vi "App - analyze RUS V6.vi"() -> ()   [LabVIEW 2018] (continued)
"radius"=0.4754648959407264}}, "timestamp(min)"=862.4166666641831, "timestamp"=timestamp(3493779566 s since 1904-01-01), "Magn Field(T)"=0.0}, {"temperature"=77.512, "lorentzian"={"A (VHz)"=0.00029695540647974435, "f (Hz)"=665.0338682665438, "G (Hz)"=0.032873121586090105, "phi(rad)"=3.411171742356422, "Q"=20230.323017085953, "Norm  Ampl"=0.015527303955909932, "bg (V)"=0.1217964163037196-0.45928093647211954i, "4corners"={"z (-pi/2)"=-0.45928093647211954-0.1297964163037196i, "z(inf)"=0.1217964163037196-0.45928093647211954i, "z (pi/2)"=0.45128093647211953+0.1217964163037196i, "z center"=-0.0040000000000000036-0.0040000000000000036i, "z(0)"=-0.1297964163037196+0.45128093647211953i, "radius"=0.4723404169344276}}, "timestamp(min)"=863.75, "timestamp"=timestamp(3493779646 s since 1904-01-01), "Magn Field(T)"=0.0}, {"temperature"=77.434, "lorentzian"={"A (VHz)"=0.0002808833623249405, "f (Hz)"=665.0132269511125, "G (Hz)"=0.030053559356176034, "phi(rad)"=3.2164772260932604, "Q"=22127.602892881696, "Norm  Ampl"=0.014704545280424244, "bg (V)"=0.05660513936673565-0.4919067745838443i, "4corners"={"z (-pi/2)"=-0.4679067745838443-0.04060513936673563i, "z(inf)"=0.05660513936673565-0.4919067745838443i, "z (pi/2)"=0.5079067745838444+0.032605139366735626i, "z center"=0.020000000000000018-0.0040000000000000036i, "z(0)"=-0.016605139366735612+0.4839067745838443i, "radius"=0.4892779955330797}}, "timestamp(min)"=865.0666666701436, "timestamp"=timestamp(3493779725 s since 1904-01-01), "Magn Field(T)"=0.0}, {"temperature"=77.354, "lorentzian"={"A (VHz)"=0.00024324022719169407, "f (Hz)"=664.9933134080237, "G (Hz)"=0.02605319858686614, "phi(rad)"=3.1017031738643666, "Q"=25524.440355790255, "Norm  Ampl"=0.01188779498495909, "bg (V)"=0.04180368485342219-0.49192630188829584i, "4corners"={"z (-pi/2)"=-0.3959263018882958-0.01780368485342211i, "z(inf)"=0.04180368485342219-0.49192630188829584i, "z (pi/2)"=0.5159263018882959-0.05419631514657784i, "z center"=0.06000000000000005-0.035999999999999976i, "z(0)"=0.07819631514657792+0.4199263018882959i, "radius"=0.4562892707904176}}, "timestamp(min)"=866.3833333328366, "timestamp"=timestamp(3493779804 s since 1904-01-01), "Magn Field(T)"=0.0}, {"temperature"=77.279, "lorentzian"={"A (VHz)"=0.0002767684428284637, "f (Hz)"=664.9763291448037, "G (Hz)"=0.03131222664140858, "phi(rad)"=3.3392624127704833, "Q"=21236.954393572625, "Norm  Ampl"=0.014856092973334787, "bg (V)"=0.09717490852872655-0.47721119114295873i, "4corners"={"z (-pi/2)"=-0.4612111911429587-0.10517490852872656i, "z(inf)"=0.09717490852872655-0.47721119114295873i, "z (pi/2)"=0.46921119114295873+0.08117490852872654i, "z center"=0.0040000000000000036-0.01200000000000001i, "z(0)"=-0.08917490852872655+0.4532111911429587i, "radius"=0.4744502249382827}}, "timestamp(min)"=867.7166666686535, "timestamp"=timestamp(3493779884 s since 1904-01-01), "Magn Field(T)"=0.0}, {"temperature"=77.2, "lorentzian"={"A (VHz)"=0.00025465138660872073, "f (Hz)"=664.9564180576857, "G (Hz)"=0.02920076503699602, "phi(rad)"=3.2865495056553193, "Q"=22771.883449464993, "Norm  Ampl"=0.013732392409333284, "bg (V)"=0.07193111188153918-0.4693429105783114i, "4corners"={"z (-pi/2)"=-0.4613429105783114-0.07193111188153918i, "z(inf)"=0.07193111188153918-0.4693429105783114i, "z (pi/2)"=0.4693429105783114+0.06393111188153917i, "z center"=0.0040000000000000036-0.0040000000000000036i, "z(0)"=-0.06393111188153917+0.4613429105783114i, "radius"=0.470275090119556}}, "timestamp(min)"=869.0333333313465, "timestamp"=timestamp(3493779963 s since 1904-01-01), "Magn Field(T)"=0.0}, {"temperature"=77.118, "lorentzian"={"A (VHz)"=0.00027838491301398664, "f (Hz)"=664.9357800881095, "G (Hz)"=0.03181971997495915, "phi(rad)"=3.269604239812998, "Q"=20896.971457052023, "Norm  Ampl"=0.015065275703701596, "bg (V)"=0.06444261324766684-0.48158323658272556i, "4corners"={"z (-pi/2)"=-0.46558323658272555-0.07244261324766685i, "z(inf)"=0.06444261324766684-0.48158323658272556i, "z (pi/2)"=0.47358323658272555+0.048442613247666834i, "z center"=0.0040000000000000036-0.01200000000000001i, "z(0)"=-0.05644261324766684+0.45758323658272554i, "radius"=0.4734572056434615}}, "timestamp(min)"=870.3500000014901, "timestamp"=timestamp(3493780042 s since 1904-01-01), "Magn Field(T)"=0.0}, {"temperature"=77.043, "lorentzian"={"A (VHz)"=0.00025512847575077615, "f (Hz)"=664.9153463888829, "G (Hz)"=0.028245509163786278, "phi(rad)"=3.1126571502773475, "Q"=23540.568609801325, "Norm  Ampl"=0.013385825226800704, "bg (V)"=0.022289093204638705-0.5017114778047216i, "4corners"={"z (-pi/2)"=-0.43771147780472147-0.0142890932046387i, "z(inf)"=0.022289093204638705-0.5017114778047216i, "z (pi/2)"=0.5097114778047216-0.04171090679536135i, "z center"=0.03600000000000003-0.028000000000000025i, "z(0)"=0.04971090679536136+0.4457114778047215i, "radius"=0.4739098576407587}}, "timestamp(min)"=871.683333337307, "timestamp"=timestamp(3493780122 s since 1904-01-01), "Magn Field(T)"=0.0}, {"temperature"=76.965, "lorentzian"={"A (VHz)"=0.000290950002143314, "f (Hz)"=664.8962985459169, "G (Hz)"=0.033622915172790445, "phi(rad)"=3.3360289701037327, "Q"=19775.09371596632, "Norm  Ampl"=0.015800250307514467, "bg (V)"=0.08679586668019772-0.47307013478150894i, "4corners"={"z (-pi/2)"=-0.46507013478150894-0.10279586668019773i, "z(inf)"=0.08679586668019772-0.47307013478150894i, "z (pi/2)"=0.45707013478150893+0.07879586668019771i, "z center"=-0.0040000000000000036-0.01200000000000001i, "z(0)"=-0.09479586668019772+0.4490701347815089i, "radius"=0.4699250563586146}}, "timestamp(min)"=873.0, "timestamp"=timestamp(3493780201 s since 1904-01-01), "Magn Field(T)"=0.0}, {"temperature"=76.89, "lorentzian"={"A (VHz)"=0.00027920835625752665, "f (Hz)"=664.877249248592, "G (Hz)"=0.03212210537837073, "phi(rad)"=3.306412896473442, "Q"=20698.433101345967, "Norm  Ampl"=0.015111162714631697, "bg (V)"=0.06518560735297112-0.4760534616565365i, "4corners"={"z (-pi/2)"=-0.4760534616565365-0.08918560735297114i, "z(inf)"=0.06518560735297112-0.4760534616565365i, "z (pi/2)"=0.4520534616565365+0.06518560735297112i, "z center"=-0.01200000000000001-0.01200000000000001i, "z(0)"=-0.08918560735297114+0.4520534616565365i, "radius"=0.470428775967055}}, "timestamp(min)"=874.3333333358169, "timestamp"=timestamp(3493780281 s since 1904-01-01), "Magn Field(T)"=0.0}, {"temperature"=76.811, "lorentzian"={"A (VHz)"=0.0002809182349613738, "f (Hz)"=664.8577998829521, "G (Hz)"=0.03227972899383772, "phi(rad)"=3.326321935294232, "Q"=20596.75903753328, "Norm  Ampl"=0.01526280982428019, "bg (V)"=0.09084953461030412-0.4767848365941506i, "4corners"={"z (-pi/2)"=-0.4607848365941506-0.09884953461030413i, "z(inf)"=0.09084953461030412-0.4767848365941506i, "z (pi/2)"=0.4687848365941506+0.07484953461030411i, "z center"=0.0040000000000000036-0.01200000000000001i, "z(0)"=-0.08284953461030412+0.4527848365941506i, "radius"=0.47282955278818783}}, "timestamp(min)"=875.6499999985099, "timestamp"=timestamp(3493780360 s since 1904-01-01), "Magn Field(T)"=0.0}, {"temperature"=76.733, "lorentzian"={"A (VHz)"=0.0002685357531772652, "f (Hz)"=664.8386786299899, "G (Hz)"=0.031013359018924134, "phi(rad)"=3.3158635131911067, "Q"=21437.170937347033, "Norm  Ampl"=0.014446963332719644, "bg (V)"=0.07677036203873196-0.4707745055716542i, "4corners"={"z (-pi/2)"=-0.46277450557165417-0.09277036203873197i, "z(inf)"=0.07677036203873196-0.4707745055716542i, "z (pi/2)"=0.45477450557165416+0.06877036203873195i, "z center"=-0.0040000000000000036-0.01200000000000001i, "z(0)"=-0.08477036203873196+0.44677450557165416i, "radius"=0.46583033214506714}}, "timestamp(min)"=876.9666666686535, "timestamp"=timestamp(3493780439 s since 1904-01-01), "Magn Field(T)"=0.0}, {"temperature"=76.659, "lorentzian"={"A (VHz)"=0.00027897248558761146, "f (Hz)"=664.8188133493377, "G (Hz)"=0.03153421429238599, "phi(rad)"=3.3051331613850907, "Q"=21082.460060210215, "Norm  Ampl"=0.014924965616204034, "bg (V)"=0.08105823087278374-0.4789792025319606i, "4corners"={"z (-pi/2)"=-0.46297920253196057-0.08905823087278375i, "z(inf)"=0.08105823087278374-0.4789792025319606i, "z (pi/2)"=0.4709792025319606+0.06505823087278373i, "z center"=0.0040000000000000036-0.01200000000000001i, "z(0)"=-0.07305823087278374+0.45497920253196056i, "radius"=0.47329435507158657}}, "timestamp(min)"=878.3000000044703, "timestamp"=timestamp(3493780519 s since 1904-01-01), "Magn Field(T)"=0.0}, {"temperature"=76.581, "lorentzian"={"A (VHz)"=0.00026752568867396, "f (Hz)"=664.8002015323394, "G (Hz)"=0.030925216416869468, "phi(rad)"=3.3462445900572364, "Q"=21497.02665200092, "Norm  Ampl"=0.014337767184288005, "bg (V)"=0.09822124554928835-0.4659519888305804i, "4corners"={"z (-pi/2)"=-0.4499519888305804-0.10622124554928836i, "z(inf)"=0.09822124554928835-0.4659519888305804i, "z (pi/2)"=0.4579519888305804+0.08222124554928834i, "z center"=0.0040000000000000036-0.01200000000000001i, "z(0)"=-0.09022124554928834+0.4419519888305804i, "radius"=0.4636270605520117}}, "timestamp(min)"=879.6166666671634, "timestamp"=timestamp(3493780598 s since 1904-01-01), "Magn Field(T)"=0.0}, {"temperature"=76.505, "lorentzian"={"A (VHz)"=0.00025864986819311913, "f (Hz)"=664.7795151476013, "G (Hz)"=0.029704329966046553, "phi(rad)"=3.2979485857827333, "Q"=22379.88589230848, "Norm  Ampl"=0.013903875658242268, "bg (V)"=0.07688857973420114-0.47436580247637555i, "4corners"={"z (-pi/2)"=-0.45836580247637554-0.08488857973420115i, "z(inf)"=0.07688857973420114-0.47436580247637555i, "z (pi/2)"=0.46636580247637555+0.06088857973420113i, "z center"=0.0040000000000000036-0.01200000000000001i, "z(0)"=-0.06888857973420114+0.45036580247637553i, "radius"=0.46807572074963655}}, "timestamp(min)"=880.9500000029802, "timestamp"=timestamp(3493780678 s since 1904-01-01), "Magn Field(T)"=0.0}, {"temperature"=76.428, "lorentzian"={"A (VHz)"=0.0002755418131497793, "f (Hz)"=664.7593151593608, "G (Hz)"=0.031231892673605332, "phi(rad)"=3.2953909958155867, "Q"=21284.631133519535, "Norm  Ampl"=0.014593455577151493, "bg (V)"=0.06758104109961673-0.47374592702124485i, "4corners"={"z (-pi/2)"=-0.46574592702124484-0.08358104109961674i, "z(inf)"=0.06758104109961673-0.47374592702124485i, "z (pi/2)"=0.45774592702124484+0.05958104109961672i, "z center"=-0.0040000000000000036-0.01200000000000001i, "z(0)"=-0.07558104109961673+0.44974592702124483i, "radius"=0.4672613257756454}}, "timestamp(min)"=882.2666666656733, "timestamp"=timestamp(3493780757 s since 1904-01-01), "Magn Field(T)"=0.0}, {"temperature"=76.351, "lorentzian"={"A (VHz)"=0.00026574292469974984, "f (Hz)"=664.7400281342468, "G (Hz)"=0.030457729512904052, "phi(rad)"=3.3023067874934755, "Q"=21825.00267633593, "Norm  Ampl"=0.014264746051900744, "bg (V)"=0.06294616436751165-0.4743102300273674i, "4corners"={"z (-pi/2)"=-0.4743102300273674-0.08694616436751167i, "z(inf)"=0.06294616436751165-0.4743102300273674i, "z (pi/2)"=0.45031023002736736+0.06294616436751165i, "z center"=-0.01200000000000001-0.01200000000000001i, "z(0)"=-0.08694616436751167+0.45031023002736736i, "radius"=0.4683456803914811}}, "timestamp(min)"=883.5833333358169, "timestamp"=timestamp(3493780836 s since 1904-01-01), "Magn Field(T)"=0.0}, {"temperature"=76.277, "lorentzian"={"A (VHz)"=0.0002653122550201634, "f (Hz)"=664.7196311232841, "G (Hz)"=0.03045838694481064, "phi(rad)"=3.2922998833660313, "Q"=21823.861924393077, "Norm  Ampl"=0.014185989270465337, "bg (V)"=0.0579264643836625-0.4724706462022241i, "4corners"={"z (-pi/2)"=-0.4724706462022241-0.08192646438366252i, "z(inf)"=0.0579264643836625-0.4724706462022241i, "z (pi/2)"=0.4484706462022241+0.0579264643836625i, "z center"=-0.01200000000000001-0.01200000000000001i, "z(0)"=-0.08192646438366252+0.4484706462022241i, "radius"=0.46574985392922397}}, "timestamp(min)"=884.9166666641831, "timestamp"=timestamp(3493780916 s since 1904-01-01), "Magn Field(T)"=0.0}, {"temperature"=76.2, "lorentzian"={"A (VHz)"=0.00026776979430489893, "f (Hz)"=664.7007475651434, "G (Hz)"=0.03066768438133285, "phi(rad)"=3.311925831059125, "Q"=21674.305086097105, "Norm  Ampl"=0.01441339308962391, "bg (V)"=0.07566772214884727-0.47518487085764655i, "4corners"={"z (-pi/2)"=-0.46718487085764654-0.09166772214884729i, "z(inf)"=0.07566772214884727-0.47518487085764655i, "z (pi/2)"=0.45918487085764653+0.06766772214884727i, "z center"=-0.0040000000000000036-0.01200000000000001i, "z(0)"=-0.08366772214884728+0.4511848708576465i, "radius"=0.4699863514441676}}, "timestamp(min)"=886.2333333343267, "timestamp"=timestamp(3493780995 s since 1904-01-01), "Magn Field(T)"=0.0}, {"temperature"=76.124, "lorentzian"={"A (VHz)"=0.0002520973866068134, "f (Hz)"=664.6803637054721, "G (Hz)"=0.028684551565679502, "phi(rad)"=3.2758784190989907, "Q"=23172.067451831772, "Norm  Ampl"=0.013553204498527708, "bg (V)"=0.05925835181710527-0.48023767768799197i, "4corners"={"z (-pi/2)"=-0.47223767768799196-0.07525835181710529i, "z(inf)"=0.05925835181710527-0.48023767768799197i, "z (pi/2)"=0.46423767768799196+0.051258351817105266i, "z center"=-0.0040000000000000036-0.01200000000000001i, "z(0)"=-0.06725835181710528+0.45623767768799195i, "radius"=0.4724914199022671}}, "timestamp(min)"=887.5500000044703, "timestamp"=timestamp(3493781074 s since 1904-01-01), "Magn Field(T)"=0.0}, {"temperature"=76.051, "lorentzian"={"A (VHz)"=0.00025530324968576736, "f (Hz)"=664.6597602636057, "G (Hz)"=0.029301482347429006, "phi(rad)"=3.2287016575527323, "Q"=22683.485851763562, "Norm  Ampl"=0.013750271926166796, "bg (V)"=0.03682586244131608-0.4794895405889917i, "4corners"={"z (-pi/2)"=-0.4714895405889917-0.052825862441316096i, "z(inf)"=0.03682586244131608-0.4794895405889917i, "z (pi/2)"=0.46348954058899167+0.028825862441316075i, "z center"=-0.0040000000000000036-0.01200000000000001i, "z(0)"=-0.04482586244131609+0.45548954058899166i, "radius"=0.46926881592982905}}, "timestamp(min)"=888.8833333328366, "timestamp"=timestamp(3493781154 s since 1904-01-01), "Magn Field(T)"=0.0}, {"temperature"=75.976, "lorentzian"={"A (VHz)"=0.00024264786629345106, "f (Hz)"=664.6404420947947, "G (Hz)"=0.027734595738420412, "phi(rad)"=3.2252805794751698, "Q"=23964.30971496282, "Norm  Ampl"=0.012948505445398125, "bg (V)"=0.02702595571733299-0.4772380190600956i, "4corners"={"z (-pi/2)"=-0.4772380190600956-0.05102595571733301i, "z(inf)"=0.02702595571733299-0.4772380190600956i, "z (pi/2)"=0.4532380190600956+0.02702595571733299i, "z center"=-0.01200000000000001-0.01200000000000001i, "z(0)"=-0.05102595571733301+0.4532380190600956i, "radius"=0.466871973455907}}, "timestamp(min)"=890.2000000029802, "timestamp"=timestamp(3493781233 s since 1904-01-01), "Magn Field(T)"=0.0}, {"temperature"=75.901, "lorentzian"={"A (VHz)"=0.00025702011963152935, "f (Hz)"=664.6201051910199, "G (Hz)"=0.029589667314684452, "phi(rad)"=3.2372526158024844, "Q"=22461.222632982735, "Norm  Ampl"=0.013728192772598631, "bg (V)"=0.03231399766194823-0.4738310960824186i, "4corners"={"z (-pi/2)"=-0.4738310960824186-0.05631399766194825i, "z(inf)"=0.03231399766194823-0.4738310960824186i, "z (pi/2)"=0.44983109608241856+0.03231399766194823i, "z center"=-0.01200000000000001-0.01200000000000001i, "z(0)"=-0.05631399766194825+0.44983109608241856i, "radius"=0.4639522515275374}}, "timestamp(min)"=891.5333333313465, "timestamp"=timestamp(3493781313 s since 1904-01-01), "Magn Field(T)"=0.0}, {"temperature"=75.826, "lorentzian"={"A (VHz)"=0.0002760497611584135, "f (Hz)"=664.5980460508742, "G (Hz)"=0.031198094391174443, "phi(rad)"=3.264679813128181, "Q"=21302.520523140698, "Norm  Ampl"=0.01425255477262775, "bg (V)"=0.028089325857898882-0.46538425279967466i, "4corners"={"z (-pi/2)"=-0.4813842527996747-0.06808932585789892i, "z(inf)"=0.028089325857898882-0.46538425279967466i, "z (pi/2)"=0.4253842527996746+0.044089325857898896i, "z center"=-0.028000000000000025-0.01200000000000001i, "z(0)"=-0.08408932585789894+0.44138425279967464i, "radius"=0.45684055551353236}}, "timestamp(min)"=892.8500000014901, "timestamp"=timestamp(3493781392 s since 1904-01-01), "Magn Field(T)"=0.0}, {"temperature"=75.75, "lorentzian"={"A (VHz)"=0.00024899250764678937, "f (Hz)"=664.5800253851179, "G (Hz)"=0.02830618097319679, "phi(rad)"=3.260796001766887, "Q"=23478.265259958975, "Norm  Ampl"=0.013124659537484923, "bg (V)"=0.04313993125916649-0.46437728981455684i, "4corners"={"z (-pi/2)"=-0.47237728981455684-0.05913993125916651i, "z(inf)"=0.04313993125916649-0.46437728981455684i, "z (pi/2)"=0.4483772898145568+0.0511399312591665i, "z center"=-0.01200000000000001-0.0040000000000000036i, "z(0)"=-0.06713993125916651+0.45637728981455683i, "radius"=0.4636676190939606}}, "timestamp(min)"=894.1666666641831, "timestamp"=timestamp(3493781471 s since 1904-01-01), "Magn Field(T)"=0.0}, {"temperature"=75.678, "lorentzian"={"A (VHz)"=0.0002622374955717733, "f (Hz)"=664.5603925639282, "G (Hz)"=0.02923189059225668, "phi(rad)"=3.2715193958776583, "Q"=22734.088664794246, "Norm  Ampl"=0.013827664667320543, "bg (V)"=0.06528693618699404-0.4810465230194425i, "4corners"={"z (-pi/2)"=-0.4650465230194425-0.07328693618699404i, "z(inf)"=0.06528693618699404-0.4810465230194425i, "z (pi/2)"=0.4730465230194425+0.04928693618699402i, "z center"=0.0040000000000000036-0.01200000000000001i, "z(0)"=-0.05728693618699403+0.4570465230194425i, "radius"=0.473033539301197}}, "timestamp(min)"=895.5, "timestamp"=timestamp(3493781551 s since 1904-01-01), "Magn Field(T)"=0.0}, {"temperature"=75.603, "lorentzian"={"A (VHz)"=0.00025369645376320597, "f (Hz)"=664.5418250189807, "G (Hz)"=0.02847618597296087, "phi(rad)"=3.289422359013243, "Q"=23336.756742984693, "Norm  Ampl"=0.013332067075039563, "bg (V)"=0.05695954846150056-0.47507659375339856i, "4corners"={"z (-pi/2)"=-0.47507659375339856-0.08095954846150058i, "z(inf)"=0.05695954846150056-0.47507659375339856i, "z (pi/2)"=0.45107659375339854+0.05695954846150056i, "z center"=-0.01200000000000001-0.01200000000000001i, "z(0)"=-0.08095954846150058+0.45107659375339854i, "radius"=0.46818303152321117}}, "timestamp(min)"=896.8166666701436, "timestamp"=timestamp(3493781630 s since 1904-01-01), "Magn Field(T)"=0.0}, {"temperature"=75.531, "lorentzian"={"A (VHz)"=0.00023340707593504762, "f (Hz)"=664.5225693944557, "G (Hz)"=0.02651623074638483, "phi(rad)"=3.2625310850781446, "Q"=25060.97400306623, "Norm  Ampl"=0.012400739338469526, "bg (V)"=0.05242101978124665-0.4682500920602771i, "4corners"={"z (-pi/2)"=-0.4682500920602771-0.06042101978124666i, "z(inf)"=0.05242101978124665-0.4682500920602771i, "z (pi/2)"=0.4602500920602771+0.05242101978124665i, "z center"=-0.0040000000000000036-0.0040000000000000036i, "z(0)"=-0.06042101978124666+0.4602500920602771i, "radius"=0.4676659913347683}}, "timestamp(min)"=898.1333333328366, "timestamp"=timestamp(3493781709 s since 1904-01-01), "Magn Field(T)"=0.0}, {"temperature"=75.457, "lorentzian"={"A (VHz)"=0.0002336852901965263, "f (Hz)"=664.5035369558955, "G (Hz)"=0.02636220320650127, "phi(rad)"=3.2498826582083717, "Q"=25206.6768376939, "Norm  Ampl"=0.012547234895950955, "bg (V)"=0.04744054446156901-0.4771674995657681i, "4corners"={"z (-pi/2)"=-0.4771674995657681-0.05544054446156902i, "z(inf)"=0.04744054446156901-0.4771674995657681i, "z (pi/2)"=0.4691674995657681+0.04744054446156901i, "z center"=-0.0040000000000000036-0.0040000000000000036i, "z(0)"=-0.05544054446156902+0.4691674995657681i, "radius"=0.4759554729802188}}, "timestamp(min)"=899.4666666686535, "timestamp"=timestamp(3493781789 s since 1904-01-01), "Magn Field(T)"=0.0}, {"temperature"=75.379, "lorentzian"={"A (VHz)"=0.00024153063716415095, "f (Hz)"=664.4828049621776, "G (Hz)"=0.027491243131012023, "phi(rad)"=3.2413753898993436, "Q"=24170.70780668318, "Norm  Ampl"=0.0128420217761985, "bg (V)"=0.034534334882454755-0.4768077695559386i, "4corners"={"z (-pi/2)"=-0.4768077695559386-0.058534334882454776i, "z(inf)"=0.034534334882454755-0.4768077695559386i, "z (pi/2)"=0.4528077695559386+0.034534334882454755i, "z center"=-0.01200000000000001-0.01200000000000001i, "z(0)"=-0.058534334882454776+0.4528077695559386i, "radius"=0.46713135942957096}}, "timestamp(min)"=900.7833333313465, "timestamp"=timestamp(3493781868 s since 1904-01-01), "Magn Field(T)"=0.0}, {"temperature"=75.31, "lorentzian"={"A (VHz)"=0.0002148911358422662, "f (Hz)"=664.465505288, "G (Hz)"=0.0249892411708139, "phi(rad)"=3.230164637465835, "Q"=26590.063329496388, "Norm  Ampl"=0.011708148514720532, "bg (V)"=0.029444178758426018-0.4706909755154814i, "4corners"={"z (-pi/2)"=-0.4786909755154814-0.04544417875842603i, "z(inf)"=0.029444178758426018-0.4706909755154814i, "z (pi/2)"=0.4546909755154814+0.037444178758426025i, "z center"=-0.01200000000000001-0.0040000000000000036i, "z(0)"=-0.05344417875842604+0.4626909755154814i, "radius"=0.4685275729138596}}, "timestamp(min)"=902.1166666671634, "timestamp"=timestamp(3493781948 s since 1904-01-01), "Magn Field(T)"=0.0}, {"temperature"=75.236, "lorentzian"={"A (VHz)"=0.00021607881434867007, "f (Hz)"=664.4465122323005, "G (Hz)"=0.02482773012791668, "phi(rad)"=3.2228412903142463, "Q"=26762.27382885827, "Norm  Ampl"=0.011626921800788802, "bg (V)"=0.026007201380307272-0.4787589912674245i, "4corners"={"z (-pi/2)"=-0.4787589912674245-0.050007201380307294i, "z(inf)"=0.026007201380307272-0.4787589912674245i, "z (pi/2)"=0.4547589912674245+0.026007201380307272i, "z center"=-0.01200000000000001-0.01200000000000001i, "z(0)"=-0.050007201380307294+0.4547589912674245i, "radius"=0.4683038578591328}}, "timestamp(min)"=903.433333337307, "timestamp"=timestamp(3493782027 s since 1904-01-01), "Magn Field(T)"=0.0}, {"temperature"=75.165, "lorentzian"={"A (VHz)"=0.00022778316000829723, "f (Hz)"=664.4269581428752, "G (Hz)"=0.02616172058956767, "phi(rad)"=3.18968018527854, "Q"=25396.913626843954, "Norm  Ampl"=0.01215429693957177, "bg (V)"=0.0023320521845758245-0.4760461907934517i, "4corners"={"z (-pi/2)"=-0.4840461907934517-0.034332052184575856i, "z(inf)"=0.0023320521845758245-0.4760461907934517i, "z (pi/2)"=0.44404619079345165+0.010332052184575832i, "z center"=-0.020000000000000018-0.01200000000000001i, "z(0)"=-0.042332052184575863+0.45204619079345165i, "radius"=0.4645832409210293}}, "timestamp(min)"=904.75, "timestamp"=timestamp(3493782106 s since 1904-01-01), "Magn Field(T)"=0.0}, {"temperature"=75.09, "lorentzian"={"A (VHz)"=0.00021406840846822526, "f (Hz)"=664.4071198861543, "G (Hz)"=0.024994078560984633, "phi(rad)"=3.171877949844509, "Q"=26582.5810807558, "Norm  Ampl"=0.010524901202167375, "bg (V)"=-0.047248938733693534-0.4249026882143163i, "4corners"={"z (-pi/2)"=-0.4809026882143163-0.016751061266306468i, "z(inf)"=-0.047248938733693534-0.4249026882143163i, "z (pi/2)"=0.3609026882143163+0.008751061266306459i, "z center"=-0.06-0.0040000000000000036i, "z(0)"=-0.07275106126630645+0.4169026882143163i, "radius"=0.42109578780778023}}, "timestamp(min)"=906.0833333358169, "timestamp"=timestamp(3493782186 s since 1904-01-01), "Magn Field(T)"=0.0}, {"temperature"=75.015, "lorentzian"={"A (VHz)"=0.00022681346010083628, "f (Hz)"=664.3873432834985, "G (Hz)"=0.026628930725100308, "phi(rad)"=3.201301138391085, "Q"=24949.831825475816, "Norm  Ampl"=0.011553536611108126, "bg (V)"=-0.026109574618153927-0.4370984249069626i, "4corners"={"z (-pi/2)"=-0.4850984249069626-0.029890425381846067i, "z(inf)"=-0.026109574618153927-0.4370984249069626i, "z (pi/2)"=0.3810984249069626+0.02189042538184606i, "z center"=-0.05199999999999999-0.0040000000000000036i, "z(0)"=-0.07789042538184605+0.4290984249069626i, "radius"=0.4338715936580141}}, "timestamp(min)"=907.3999999985099, "timestamp"=timestamp(3493782265 s since 1904-01-01), "Magn Field(T)"=0.0}, {"temperature"=74.945, "lorentzian"={"A (VHz)"=0.00023488220890380816, "f (Hz)"=664.3683940302727, "G (Hz)"=0.027425386022977043, "phi(rad)"=3.2232642890579752, "Q"=24224.577676816054, "Norm  Ampl"=0.012190055722490472, "bg (V)"=-0.007738874706385353-0.45499915812940217i, "4corners"={"z (-pi/2)"=-0.48699915812940214-0.04826112529361464i, "z(inf)"=-0.007738874706385353-0.45499915812940217i, "z (pi/2)"=0.3989991581294022+0.02426112529361462i, "z center"=-0.043999999999999984-0.01200000000000001i, "z(0)"=-0.08026112529361462+0.43099915812940215i, "radius"=0.4444807344654189}}, "timestamp(min)"=908.7333333343267, "timestamp"=timestamp(3493782345 s since 1904-01-01), "Magn Field(T)"=0.0}, {"temperature"=74.872, "lorentzian"={"A (VHz)"=0.00023255713109856803, "f (Hz)"=664.3480022893341, "G (Hz)"=0.027106611066603756, "phi(rad)"=3.2084285772770182, "Q"=24508.70751260503, "Norm  Ampl"=0.011232234566965142, "bg (V)"=-0.0403256447807529-0.41744734878375084i, "4corners"={"z (-pi/2)"=-0.48144734878375084-0.03167435521924711i, "z(inf)"=-0.0403256447807529-0.41744734878375084i, "z (pi/2)"=0.34544734878375083+0.0236743552192471i, "z center"=-0.068-0.0040000000000000036i, "z(0)"=-0.09567435521924711+0.40944734878375083i, "radius"=0.41437251375195433}}, "timestamp(min)"=910.0500000044703, "timestamp"=timestamp(3493782424 s since 1904-01-01), "Magn Field(T)"=0.0}, {"temperature"=74.801, "lorentzian"={"A (VHz)"=0.00023198701093833003, "f (Hz)"=664.3290848387534, "G (Hz)"=0.027392543809990896, "phi(rad)"=3.238350736893019, "Q"=24252.186633227262, "Norm  Ampl"=0.012931296054372234, "bg (V)"=0.03360569533601324-0.48186549109289656i, "4corners"={"z (-pi/2)"=-0.48186549109289656-0.057605695336013264i, "z(inf)"=0.03360569533601324-0.48186549109289656i, "z (pi/2)"=0.45786549109289654+0.03360569533601324i, "z center"=-0.01200000000000001-0.01200000000000001i, "z(0)"=-0.057605695336013264+0.45786549109289654i, "radius"=0.4720735738918777}}, "timestamp(min)"=911.3666666671634, "timestamp"=timestamp(3493782503 s since 1904-01-01), "Magn Field(T)"=0.0}, {"temperature"=74.729, "lorentzian"={"A (VHz)"=0.0002134569187991555, "f (Hz)"=664.3099632939094, "G (Hz)"=0.025270654278756556, "phi(rad)"=3.2035288612614794, "Q"=26287.802285054124, "Norm  Ampl"=0.011634964964844275, "bg (V)"=0.008498073516200383-0.46353126346544293i, "4corners"={"z (-pi/2)"=-0.47953126346544295-0.032498073516200404i, "z(inf)"=0.008498073516200383-0.46353126346544293i, "z (pi/2)"=0.4395312634654429+0.024498073516200397i, "z center"=-0.020000000000000018-0.0040000000000000036i, "z(0)"=-0.04849807351620042+0.4555312634654429i, "radius"=0.4604140769962199}}, "timestamp(min)"=912.7000000029802, "timestamp"=timestamp(3493782583 s since 1904-01-01), "Magn Field(T)"=0.0}, {"temperature"=74.657, "lorentzian"={"A (VHz)"=0.00021496379655795716, "f (Hz)"=664.2898717746746, "G (Hz)"=0.025574849608406777, "phi(rad)"=3.207228129778737, "Q"=25974.341274574457, "Norm  Ampl"=0.011077101095142637, "bg (V)"=-0.015592056088489615-0.4441921601135659i, "4corners"={"z (-pi/2)"=-0.47619216011356585-0.04040794391151038i, "z(inf)"=-0.015592056088489615-0.4441921601135659i, "z (pi/2)"=0.3881921601135659+0.016407943911510358i, "z center"=-0.043999999999999984-0.01200000000000001i, "z(0)"=-0.07240794391151036+0.42019216011356586i, "radius"=0.4331247794122494}}, "timestamp(min)"=914.0166666656733, "timestamp"=timestamp(3493782662 s since 1904-01-01), "Magn Field(T)"=0.0}, {"temperature"=74.584, "lorentzian"={"A (VHz)"=0.00021328480237914658, "f (Hz)"=664.2707763707501, "G (Hz)"=0.024915785937746585, "phi(rad)"=3.1758437835330815, "Q"=26660.639083610124, "Norm  Ampl"=0.010058255175399333, "bg (V)"=-0.062175862533385126-0.41545329290542443i, "4corners"={"z (-pi/2)"=-0.47945329290542443-0.025824137466614897i, "z(inf)"=-0.062175862533385126-0.41545329290542443i, "z (pi/2)"=0.3274532929054244+0.0018241374666148735i, "z center"=-0.07600000000000001-0.01200000000000001i, "z(0)"=-0.0898241374666149+0.3914532929054244i, "radius"=0.40369006221719905}}, "timestamp(min)"=915.3333333358169, "timestamp"=timestamp(3493782741 s since 1904-01-01), "Magn Field(T)"=0.0}, {"temperature"=74.514, "lorentzian"={"A (VHz)"=0.00018772288676282073, "f (Hz)"=664.2525985561252, "G (Hz)"=0.022142380285421964, "phi(rad)"=3.1504427140832316, "Q"=29999.150497539504, "Norm  Ampl"=0.010077477654590583, "bg (V)"=-0.02397219804339326-0.4591038720884046i, "4corners"={"z (-pi/2)"=-0.4831038720884046-0.008027801956606767i, "z(inf)"=-0.02397219804339326-0.4591038720884046i, "z (pi/2)"=0.42710387208840456+2.780195660676086e-05i, "z center"=-0.028000000000000025-0.0040000000000000036i, "z(0)"=-0.03202780195660679+0.4511038720884046i, "radius"=0.4551216953502223}}, "timestamp(min)"=916.6666666641831, "timestamp"=timestamp(3493782821 s since 1904-01-01), "Magn Field(T)"=0.0}, {"temperature"=74.444, "lorentzian"={"A (VHz)"=0.0001922604583890046, "f (Hz)"=664.2332987241489, "G (Hz)"=0.02293406780651738, "phi(rad)"=3.155750253511057, "Q"=28962.733708120795, "Norm  Ampl"=0.010630124865586866, "bg (V)"=-0.013438057795310562-0.4754615906129815i, "4corners"={"z (-pi/2)"=-0.4834615906129815-0.018561942204689465i, "z(inf)"=-0.013438057795310562-0.4754615906129815i, "z (pi/2)"=0.44346159061298146-0.005438057795310555i, "z center"=-0.020000000000000018-0.01200000000000001i, "z(0)"=-0.026561942204689472+0.45146159061298147i, "radius"=0.4635080420650892}}, "timestamp(min)"=917.9833333343267, "timestamp"=timestamp(3493782900 s since 1904-01-01), "Magn Field(T)"=0.0}, {"temperature"=74.37, "lorentzian"={"A (VHz)"=0.0001802693347115753, "f (Hz)"=664.2145643903633, "G (Hz)"=0.021662797023169204, "phi(rad)"=3.139385823517819, "Q"=30661.532935011117, "Norm  Ampl"=0.009185517488949907, "bg (V)"=-0.06093574526623-0.4280216585118314i, "4corners"={"z (-pi/2)"=-0.4840216585118314-0.0030642547337699977i, "z(inf)"=-0.06093574526623-0.4280216585118314i, "z (pi/2)"=0.3640216585118314-0.0049357452662300095i, "z center"=-0.06-0.0040000000000000036i, "z(0)"=-0.05906425473376999+0.4200216585118314i, "radius"=0.42402269102764706}}, "timestamp(min)"=919.3166666701436, "timestamp"=timestamp(3493782980 s since 1904-01-01), "Magn Field(T)"=0.0}, {"temperature"=74.299, "lorentzian"={"A (VHz)"=0.00018314419547672513, "f (Hz)"=664.1958790605045, "G (Hz)"=0.021819903597934308, "phi(rad)"=3.1341852457674895, "Q"=30439.908961072768, "Norm  Ampl"=0.00895972782128557, "bg (V)"=-0.0710416152261022-0.4146105223357084i, "4corners"={"z (-pi/2)"=-0.4786105223357084-0.000958384773897814i, "z(inf)"=-0.0710416152261022-0.4146105223357084i, "z (pi/2)"=0.3426105223357084-0.007041615226102194i, "z center"=-0.068-0.0040000000000000036i, "z(0)"=-0.06495838477389781+0.4066105223357084i, "radius"=0.41062178762942786}}, "timestamp(min)"=920.6333333328366, "timestamp"=timestamp(3493783059 s since 1904-01-01), "Magn Field(T)"=0.0}, {"temperature"=74.229, "lorentzian"={"A (VHz)"=0.00019027847592443438, "f (Hz)"=664.17627848522, "G (Hz)"=0.022575581161975403, "phi(rad)"=3.1179021402025535, "Q"=29420.118743339735, "Norm  Ampl"=0.008733513636959029, "bg (V)"=-0.10116397532445093-0.39074809248481873i, "4corners"={"z (-pi/2)"=-0.47874809248481875+0.005163975324450905i, "z(inf)"=-0.10116397532445093-0.39074809248481873i, "z (pi/2)"=0.2947480924848187-0.013163975324450912i, "z center"=-0.09200000000000003-0.0040000000000000036i, "z(0)"=-0.08283602467554912+0.3827480924848187i, "radius"=0.3868566472020263}}, "timestamp(min)"=921.9500000029802, "timestamp"=timestamp(3493783138 s since 1904-01-01), "Magn Field(T)"=0.0}, {"temperature"=74.159, "lorentzian"={"A (VHz)"=0.00019094203357565123, "f (Hz)"=664.1574446299836, "G (Hz)"=0.022818580126552277, "phi(rad)"=3.1456512996482813, "Q"=29105.993490679695, "Norm  Ampl"=0.008825574923115868, "bg (V)"=-0.09043023595964923-0.3907682469352591i, "4corners"={"z (-pi/2)"=-0.4787682469352591-0.005569764040350798i, "z(inf)"=-0.09043023595964923-0.3907682469352591i, "z (pi/2)"=0.29476824693525905-0.0024302359596492093i, "z center"=-0.09200000000000003-0.0040000000000000036i, "z(0)"=-0.09356976404035082+0.38276824693525907i, "radius"=0.38677143249794954}}, "timestamp(min)"=923.2833333313465, "timestamp"=timestamp(3493783218 s since 1904-01-01), "Magn Field(T)"=0.0}, {"temperature"=74.09, "lorentzian"={"A (VHz)"=0.00020596834323652265, "f (Hz)"=664.1383117517026, "G (Hz)"=0.02449055404845634, "phi(rad)"=3.1729776932137916, "Q"=27118.14156746543, "Norm  Ampl"=0.010071352863495161, "bg (V)"=-0.05509551780180038-0.4230316575583201i, "4corners"={"z (-pi/2)"=-0.4790316575583201-0.024904482198199636i, "z(inf)"=-0.05509551780180038-0.4230316575583201i, "z (pi/2)"=0.3430316575583201+0.0009044821981996163i, "z center"=-0.068-0.01200000000000001i, "z(0)"=-0.08090448219819964+0.3990316575583201i, "radius"=0.4112341780250564}}, "timestamp(min)"=924.6000000014901, "timestamp"=timestamp(3493783297 s since 1904-01-01), "Magn Field(T)"=0.0}, {"temperature"=74.017, "lorentzian"={"A (VHz)"=0.00019600856760996083, "f (Hz)"=664.1189516478559, "G (Hz)"=0.02319843186355, "phi(rad)"=3.1525043729887807, "Q"=28627.751890908512, "Norm  Ampl"=0.009533839941620222, "bg (V)"=-0.0635157088870945-0.41494468915149957i, "4corners"={"z (-pi/2)"=-0.47894468915149957-0.008484291112905506i, "z(inf)"=-0.0635157088870945-0.41494468915149957i, "z (pi/2)"=0.34294468915149956+0.00048429111290549786i, "z center"=-0.068-0.0040000000000000036i, "z(0)"=-0.07248429111290551+0.40694468915149956i, "radius"=0.41096915505741777}}, "timestamp(min)"=925.9166666641831, "timestamp"=timestamp(3493783376 s since 1904-01-01), "Magn Field(T)"=0.0}, {"temperature"=73.949, "lorentzian"={"A (VHz)"=0.0001944683662669622, "f (Hz)"=664.0996935583665, "G (Hz)"=0.023276846752517517, "phi(rad)"=3.1492621517073305, "Q"=28530.48355815379, "Norm  Ampl"=0.009011010494496275, "bg (V)"=-0.08903098743399736-0.39911194743718154i, "4corners"={"z (-pi/2)"=-0.47911194743718155-0.014969012566002676i, "z(inf)"=-0.08903098743399736-0.39911194743718154i, "z (pi/2)"=0.2951119474371815-0.009030987433997346i, "z center"=-0.09200000000000003-0.01200000000000001i, "z(0)"=-0.0949690125660027+0.3751119474371815i, "radius"=0.38712333291113343}}, "timestamp(min)"=927.25, "timestamp"=timestamp(3493783456 s since 1904-01-01), "Magn Field(T)"=0.0}, {"temperature"=73.879, "lorentzian"={"A (VHz)"=0.00019439596687335025, "f (Hz)"=664.0810745610588, "G (Hz)"=0.0228019332048808, "phi(rad)"=3.1435440095658205, "Q"=29123.893513507483, "Norm  Ampl"=0.00873345297549396, "bg (V)"=-0.09125260438724586-0.3950129783053545i, "4corners"={"z (-pi/2)"=-0.4750129783053545-0.01274739561275418i, "z(inf)"=-0.09125260438724586-0.3950129783053545i, "z (pi/2)"=0.29101297830535444-0.01125260438724584i, "z center"=-0.09200000000000003-0.01200000000000001i, "z(0)"=-0.09274739561275419+0.37101297830535446i, "radius"=0.3830137075230336}}, "timestamp(min)"=928.5666666701436, "timestamp"=timestamp(3493783535 s since 1904-01-01), "Magn Field(T)"=0.0}, {"temperature"=73.808, "lorentzian"={"A (VHz)"=0.00017826308821993812, "f (Hz)"=664.0621135285246, "G (Hz)"=0.021133873033784428, "phi(rad)"=3.142723173327675, "Q"=31421.6950422178, "Norm  Ampl"=0.00857689951606022, "bg (V)"=-0.07554119379293195-0.41783635670517916i, "4corners"={"z (-pi/2)"=-0.48183635670517916-0.012458806207068077i, "z(inf)"=-0.07554119379293195-0.41783635670517916i, "z (pi/2)"=0.32983635670517913-0.011541193792931944i, "z center"=-0.07600000000000001-0.01200000000000001i, "z(0)"=-0.07645880620706808+0.39383635670517914i, "radius"=0.40583661604994326}}, "timestamp(min)"=929.8999999985099, "timestamp"=timestamp(3493783615 s since 1904-01-01), "Magn Field(T)"=0.0}, {"temperature"=73.74, "lorentzian"={"A (VHz)"=0.00016488901710533672, "f (Hz)"=664.0435393826916, "G (Hz)"=0.019647103309939264, "phi(rad)"=3.110147475046193, "Q"=33798.5467326758, "Norm  Ampl"=0.007634388028594628, "bg (V)"=-0.10421682047312142-0.4003836604628278i, "4corners"={"z (-pi/2)"=-0.4803836604628278+0.00021682047312138186i, "z(inf)"=-0.10421682047312142-0.4003836604628278i, "z (pi/2)"=0.29638366046282777-0.024216820473121403i, "z center"=-0.09200000000000003-0.01200000000000001i, "z(0)"=-0.07978317952687863+0.3763836604628278i, "radius"=0.3885757563422834}}, "timestamp(min)"=931.2166666686535, "timestamp"=timestamp(3493783694 s since 1904-01-01), "Magn Field(T)"=0.0}, {"temperature"=73.67, "lorentzian"={"A (VHz)"=0.00015214771278851755, "f (Hz)"=664.0255098851464, "G (Hz)"=0.018070863218509033, "phi(rad)"=3.0882359044209995, "Q"=36745.64418179094, "Norm  Ampl"=0.006771358404597865, "bg (V)"=-0.1279838967107916-0.37817813276316264i, "4corners"={"z (-pi/2)"=-0.4821781327631626+0.015983896710791617i, "z(inf)"=-0.1279838967107916-0.37817813276316264i, "z (pi/2)"=0.26617813276316266-0.023983896710791625i, "z center"=-0.10799999999999998-0.0040000000000000036i, "z(0)"=-0.08801610328920836+0.37017813276316264i, "radius"=0.3747113971657048}}, "timestamp(min)"=932.5333333313465, "timestamp"=timestamp(3493783773 s since 1904-01-01), "Magn Field(T)"=0.0}, {"temperature"=73.599, "lorentzian"={"A (VHz)"=0.0001427980228670688, "f (Hz)"=664.0073679349201, "G (Hz)"=0.0172513749980997, "phi(rad)"=3.027819698418239, "Q"=38490.11270162888, "Norm  Ampl"=0.006207590848793478, "bg (V)"=-0.1568508468555807-0.3615052861071481i, "4corners"={"z (-pi/2)"=-0.4735052861071481+0.036850846855580696i, "z(inf)"=-0.1568508468555807-0.3615052861071481i, "z (pi/2)"=0.2415052861071481-0.0448508468555807i, "z center"=-0.11599999999999999-0.0040000000000000036i, "z(0)"=-0.07514915314441929+0.3535052861071481i, "radius"=0.359831656866613}}, "timestamp(min)"=933.8666666671634, "timestamp"=timestamp(3493783853 s since 1904-01-01), "Magn Field(T)"=0.0}, {"temperature"=73.53, "lorentzian"={"A (VHz)"=0.0001373340077936225, "f (Hz)"=663.9886506388516, "G (Hz)"=0.016752772274285566, "phi(rad)"=3.029558938647277, "Q"=39634.553599109786, "Norm  Ampl"=0.0062292336173589615, "bg (V)"=-0.14157074221409405-0.37350190154724705i, "4corners"={"z (-pi/2)"=-0.469501901547247+0.03757074221409406i, "z(inf)"=-0.14157074221409405-0.37350190154724705i, "z (pi/2)"=0.26950190154724707-0.045570742214094066i, "z center"=-0.09999999999999998-0.0040000000000000036i, "z(0)"=-0.058429257785905915+0.36550190154724704i, "radius"=0.37183300264401237}}, "timestamp(min)"=935.183333337307, "timestamp"=timestamp(3493783932 s since 1904-01-01), "Magn Field(T)"=0.0}, {"temperature"=73.459, "lorentzian"={"A (VHz)"=0.00015716000169145204, "f (Hz)"=663.9687076319055, "G (Hz)"=0.018485551246975856, "phi(rad)"=3.036824244495425, "Q"=35918.253059428105, "Norm  Ampl"=0.006172688423615892, "bg (V)"=-0.1749202632030002-0.3440886842210592i, "4corners"={"z (-pi/2)"=-0.4720886842210592+0.022920263203000182i, "z(inf)"=-0.1749202632030002-0.3440886842210592i, "z (pi/2)"=0.19208868422105918-0.046920263203000204i, "z center"=-0.14-0.01200000000000001i, "z(0)"=-0.10507973679699982+0.3200886842210592i, "radius"=0.3339196295066242}}, "timestamp(min)"=936.5, "timestamp"=timestamp(3493784011 s since 1904-01-01), "Magn Field(T)"=0.0}, {"temperature"=73.392, "lorentzian"={"A (VHz)"=0.00017627744224923487, "f (Hz)"=663.9499123640444, "G (Hz)"=0.020780394913589104, "phi(rad)"=3.0583951364497803, "Q"=31950.78414654487, "Norm  Ampl"=0.006219372120082306, "bg (V)"=-0.19687149994830724-0.31025515108630497i, "4corners"={"z (-pi/2)"=-0.47025515108630495+0.012871499948307257i, "z(inf)"=-0.19687149994830724-0.31025515108630497i, "z (pi/2)"=0.12625515108630497-0.03687149994830728i, "z center"=-0.172-0.01200000000000001i, "z(0)"=-0.14712850005169273+0.28625515108630495i, "radius"=0.29929037181171275}}, "timestamp(min)"=937.8333333358169, "timestamp"=timestamp(3493784091 s since 1904-01-01), "Magn Field(T)"=0.0}, {"temperature"=73.325, "lorentzian"={"A (VHz)"=0.0001735579927308951, "f (Hz)"=663.9300692915438, "G (Hz)"=0.02079678127234013, "phi(rad)"=3.0483689500573607, "Q"=31924.655099131884, "Norm  Ampl"=0.0072958662795648815, "bg (V)"=-0.1566571183741111-0.36129377749056607i, "4corners"={"z (-pi/2)"=-0.47329377749056606+0.020657118374111084i, "z(inf)"=-0.1566571183741111-0.36129377749056607i, "z (pi/2)"=0.22529377749056606-0.044657118374111106i, "z center"=-0.124-0.01200000000000001i, "z(0)"=-0.09134288162588891+0.33729377749056605i, "radius"=0.35081708962667396}}, "timestamp(min)"=939.1499999985099, "timestamp"=timestamp(3493784170 s since 1904-01-01), "Magn Field(T)"=0.0}, {"temperature"=73.253, "lorentzian"={"A (VHz)"=0.00019495658027975842, "f (Hz)"=663.9104025268014, "G (Hz)"=0.023023745131469733, "phi(rad)"=3.131685954619118, 
